vi "Get Rx Hardware Channel Data.vi"(8 "error in":errorcluster, 11 "custom device ref in":T9 format="%.0x") -> (0 "error out":errorcluster, 2 "Rx hardware channel data":T1[](array[typedef]) {"labels settings for RT"."Label Timestamp Channel Data Reference" format="%.0x"; "labels settings for RT"."Word Initial Raw Value" format="%032.0f"; "labels settings for RT"."Label Disable/Trigger Channel Reference" format="%.0x"; "labels settings for RT"."parameter driver data"."Tx parameter refs" format="%.0x"; "labels settings for RT"."parameter driver data"."Rx block data refs"."Data Reference" format="%.0x"; "labels settings for RT"."SDI" format="%02b"; "labels settings for RT"."label" format="%.0o"}, 3 "custom device ref out":T9 format="%.0x")   [LabVIEW 2020]
uses:
  <vilib>/NI VeriStand/Custom Device API/Custom Device Item Ref.ctl
  RT Hardware Channel Settings.ctl
  RT Label Settings.ctl
  Label.ctl
  RT Parameters.ctl
  Parameter Definition.ctl
  Encoding and Decoding/Encoding.ctl
  <vilib>/NI VeriStand/Custom Device API/Block Data Reference.ctl
  <vilib>/NI VeriStand/Custom Device API/Data Reference.ctl
  Transfer Type.ctl
  <vilib>/NI VeriStand/Custom Device API/Data Access Type.ctl
  <vilib>/NI VeriStand/Custom Device API/Custom Device API.lvlib
  Scripting/Communication Bus Template Scripting.lvlib
  Encoding and Decoding/Encoding and Decoding.lvlib
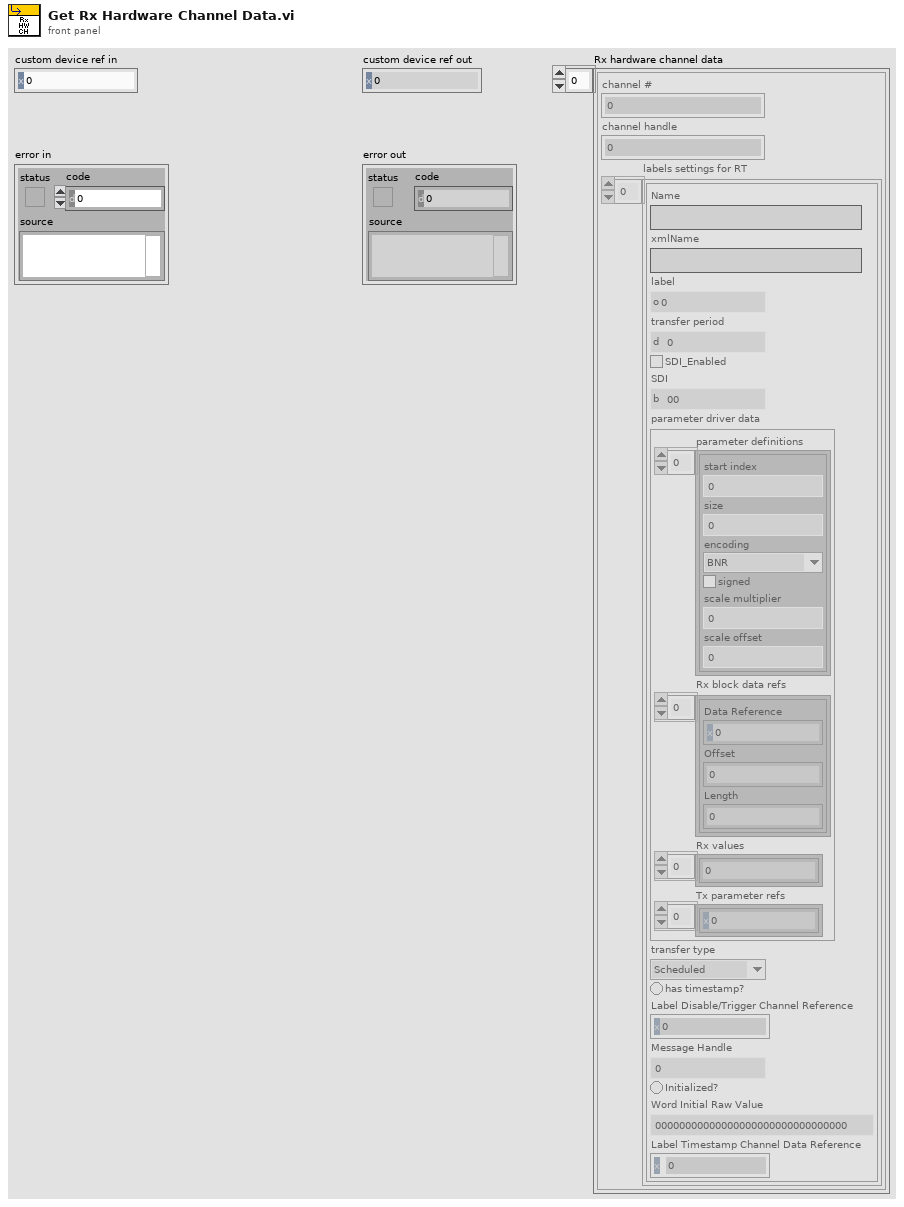
[diagram p1: front panel]
types:
  T1 = typedef "RT Hardware Channel Settings.ctl" = cluster{"channel #":u16, "channel handle":u64, "labels settings for RT":T2[]}
  T2 = typedef "RT Label Settings.ctl" = cluster{"Name":string, "xmlName":string, "label":T3, "transfer period":u32, "SDI_Enabled":bool, "SDI":u8, "parameter driver data":T4, "transfer type":T10, "has timestamp?":bool, "Label Disable/Trigger Channel Reference":T9, "Message Handle":u64, "Initialized?":bool, "Word Initial Raw Value":u32, "Label Timestamp Channel Data Reference":T8}
  T3 = typedef "Label.ctl" = u8
  T4 = typedef "RT Parameters.ctl" = cluster{"parameter definitions":T5[], "Rx block data refs":T7[], "Rx values":dbl[], "Tx parameter refs":T9[]}
  T5 = typedef "Parameter Definition.ctl" = cluster{"start index":i32, "size":i32, "encoding":T6, "signed":bool, "scale multiplier":dbl, "scale offset":dbl}
  T6 = typedef "Encoding and Decoding.lvlib/Encoding.ctl" = enum16{"BNR", "BCD", "Discrete"}
  T7 = typedef "Custom Device API.lvlib/Block Data Reference.ctl" = cluster{"Data Reference":T8, "Offset":u64, "Length":u64}
  T8 = typedef "Custom Device API.lvlib/Data Reference.ctl" = i32
  T9 = typedef "Custom Device API.lvlib/Custom Device Item Ref.ctl" = u64
  T10 = typedef "Transfer Type.ctl" = enum16{"Scheduled", "Acyclic", "Block", "Strobe"}
  T11 = typedef "Custom Device API.lvlib/Data Access Type.ctl" = enum16{"Read", "Write"}
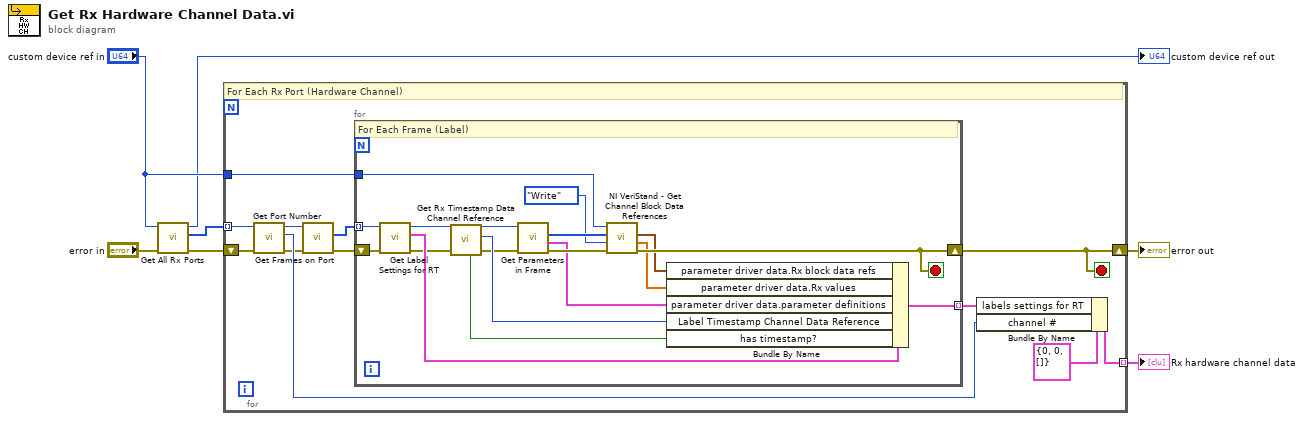
[diagram p0: block diagram]
diagram:
  n1 = call "Get All Rx Ports.vi"("error in"="error in", "Ballard ARINC 429 custom device in"="custom device ref in") -> ("error out"=w4:errorcluster, "Rx port refs"=w3:T9[], "Ballard ARINC 429 custom device out"=→"custom device ref out":T9)  [unwired: 7 in]
  n2 = for {
    tunnel: "custom device ref in" -> [w19]
    shift-right: [w18] -> w6
    shift-left: w4 -> [w13]
    tunnel: w3 -> [w14] mode=indexing
    tunnel: [w17] -> w5 mode=indexing
    stop <- w18 stop-if-true
    # "For Each Rx Port (Hardware Channel)"
    n3 = call "Get Port Number.vi"("error in"=w13, "port ref in"=w14) -> ("error out"=w10:errorcluster, "port number"=w12:u16, "port ref out"=w11:T9)  [unwired: 6 in, 1 out]
    n4 = call "Get Frames on Port.vi"("error in"=w10, "port ref in"=w11) -> ("error out"=w8:errorcluster, "frame references"=w9:T9[])  [unwired: 6 in, 2 out]
    n5 = for {
      tunnel: w9 -> [w36] mode=indexing
      tunnel: w19 -> [w30]
      shift-right: [w26] -> w18
      shift-left: w8 -> [w35]
      tunnel: [w20] -> w16 mode=indexing
      stop <- w26 stop-if-true
      # "For Each Frame (Label)"
      n6 = call "Get Label Settings for RT.vi"("error in"=w35, "label ref in"=w36) -> ("error out"=w31:errorcluster, "label settings for RT"=w33:T2, "label ref out"=w25:T9)  [unwired: 7 in]
      n7 = call "Get Rx Timestamp Data Channel Reference.vi"("error in"=w31, "frame ref in"=w25) -> ("error out"=w28:errorcluster, "timestamp channel data reference"=w29:T8, "frame ref out"=w27:T9, "timestamp channel found?"=w24:bool)  [unwired: 6 in]
      n8 = call "Get Parameters in Frame.vi"("error in"=w28, "frame ref in"=w27) -> ("error out"=w34:errorcluster, "parameter definitions"=w32:T5[], "parameter references"=w37:T9[])  [unwired: 6 in, 1 out]
      n9 = call <vilib>:"NI VeriStand - Get Channel Block Data References.vi"("error in (no error)"=w34, "Access"=Data_Access_Type."Write", "Channel Refs"=w37, "Device Ref in"=w30) -> ("error out"=w26:errorcluster, "Values Array"=w22:dbl[], "Block Data Refs"=w21:T7[])  [unwired: 4 in, 1 out]
      n10 = Bundle By Name(cluster=w33, "parameter driver data.Rx block data refs"=w21, "parameter driver data.Rx values"=w22, "parameter driver data.parameter definitions"=w32, "Label Timestamp Channel Data Reference"=w29, "has timestamp?"=w24) -> (w20:T2)
    }
    n11 = Bundle By Name(cluster=T1 {"channel #"=0, "channel handle"=0, "labels settings for RT"=[]} ("RT hardware channel"), "labels settings for RT"=w16, "channel #"=w12) -> (w17:T1)
  }
  "error out" <- w6
  "Rx hardware channel data" <- w5
